vi "serialization tests.vi"() -> ()   [LabVIEW 2013, in "sample module tests.lvlib"]
uses:
  sample module tests.lvlib
  module/configuration/sample module configuration.lvclass
panel:
  out "data":string
  out "channels equal":bool
  out "keine error":errorcluster
  out "no error":errorcluster
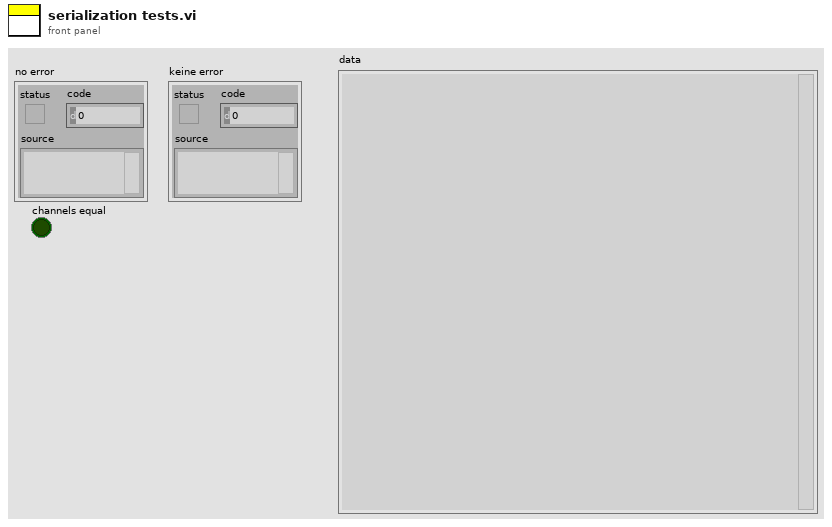
[diagram p1: front panel]
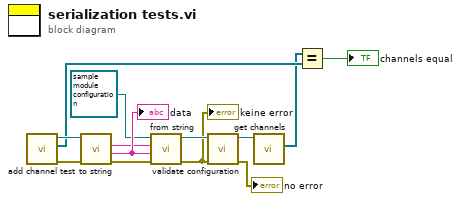
[diagram p0: block diagram]
diagram:
  n1 = call "add channel test.vi"() -> ("no error"=w4:errorcluster, "channels"=w3:refnum<class "TBM channel.lvclass">[], "sample module configuration out"=w6:refnum<class "sample module configuration.lvclass">)  [unwired: 8 in, 1 out]
  n2 = call-dynamic "to string.vi"("error in"=w4, "sample module configuration in"=w6) -> ("error out"=w13:errorcluster, "data"=w12:string, "version"=w11:string)  [unwired: 6 in, 1 out]
  "data" <- w12
  n3 = call-dynamic "from string.vi"("error in"=w13, "data"=w12, "version"=w11, "sample module configuration in"=refnum<class "sample module configuration.lvclass"> refnum ("sample module configuration Out")) -> ("error out"=w8:errorcluster, "sample module configuration out"=w10:refnum<class "sample module configuration.lvclass">)  [unwired: 6 in]
  "keine error" <- w8
  n4 = call-dynamic "validate configuration.vi"("error in"=w8, "sample module configuration in"=w10) -> ("error out"=→"no error":errorcluster, "sample module configuration out"=w2:refnum<class "sample module configuration.lvclass">)  [unwired: 8 in]
  n5 = call-dynamic "get channels.vi"("module configuration in"=w2) -> ("channels"=w1:refnum<class "TBM channel.lvclass">[])  [unwired: 9 in, 1 out]
  n6 = Equal?(x=w1, y=w3) -> (x = y?=→"channels equal":bool)
